vi "svc_Weighting to Weighting Label.vi"(9 "include weighting if dB On False (T)":bool=TRUE, 10 "dB On (T)":bool=TRUE, 11 "weighting filter":T1 items=["Linear", "A-weighting", "B-weighting", "C-weighting", "ITU-R 468-4", "Dolby", "CCITT", "C-message", "Wb", "Wc", "Wd", "We", "Wf", "Wh", "Wj", "Wk", "Wm", "AES17 20 kHz lowpass", "AES17 40 kHz lowpass", "AES17 20 kHz highpass", "AES17 40 kHz highpass"]) -> (2 "weighting string":string, 3 "weighting enum":T1 items=["Linear", "A-weighting", "B-weighting", "C-weighting", "ITU-R 468-4", "Dolby", "CCITT", "C-message", "Wb", "Wc", "Wd", "We", "Wf", "Wh", "Wj", "Wk", "Wm", "AES17 20 kHz lowpass", "AES17 40 kHz lowpass", "AES17 20 kHz highpass", "AES17 40 kHz highpass"])   [LabVIEW 2017]
uses:
  <vilib>/addons/_NISVFA/_Shared subVIs/Controls/svc_Weighting Filter Text Ring.ctl
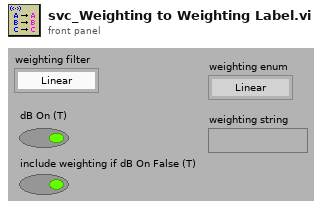
[diagram p1: front panel]
types:
  T1 = typedef "svc_Weighting Filter Text Ring.ctl" = u16
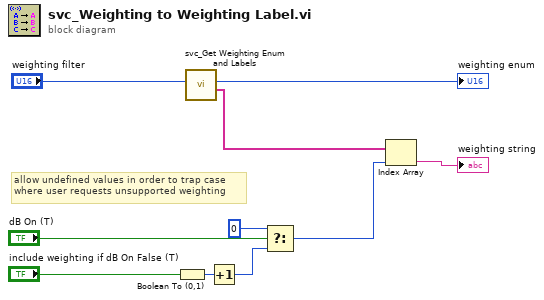
[diagram p0: block diagram]
diagram:
  # "allow undefined values in order to trap case\nwhere user requests unsupported weighting"
  n1 = Boolean To (0,1)(Boolean="include weighting if dB On False (T)") -> (0, 1=w4:i16)
  n2 = call <vilib>:"svc_Get Weighting Enum and Labels.vi"("weighting filter"="weighting filter") -> ("weighting subarray"=w8:string[], "weighting enum"=→"weighting enum":T1)  [unwired: 7 in]
  n3 = Increment(x=w4) -> (x+1=w3:i16)
  n4 = Select(t=0 ("disabled index (col)"), s="dB On (T)", f=w3) -> (s? t:f=w1:i32)
  n5 = Index Array(array=w8, index=w1) -> (element=→"weighting string":string)
